vi "Save Copy of Cal Coefficients.vi"() -> ()   [LabVIEW 2016]
uses:
  Miscellaneous/Globals.vi
panel:
  out "Spreadsheet":string[][](array[string])
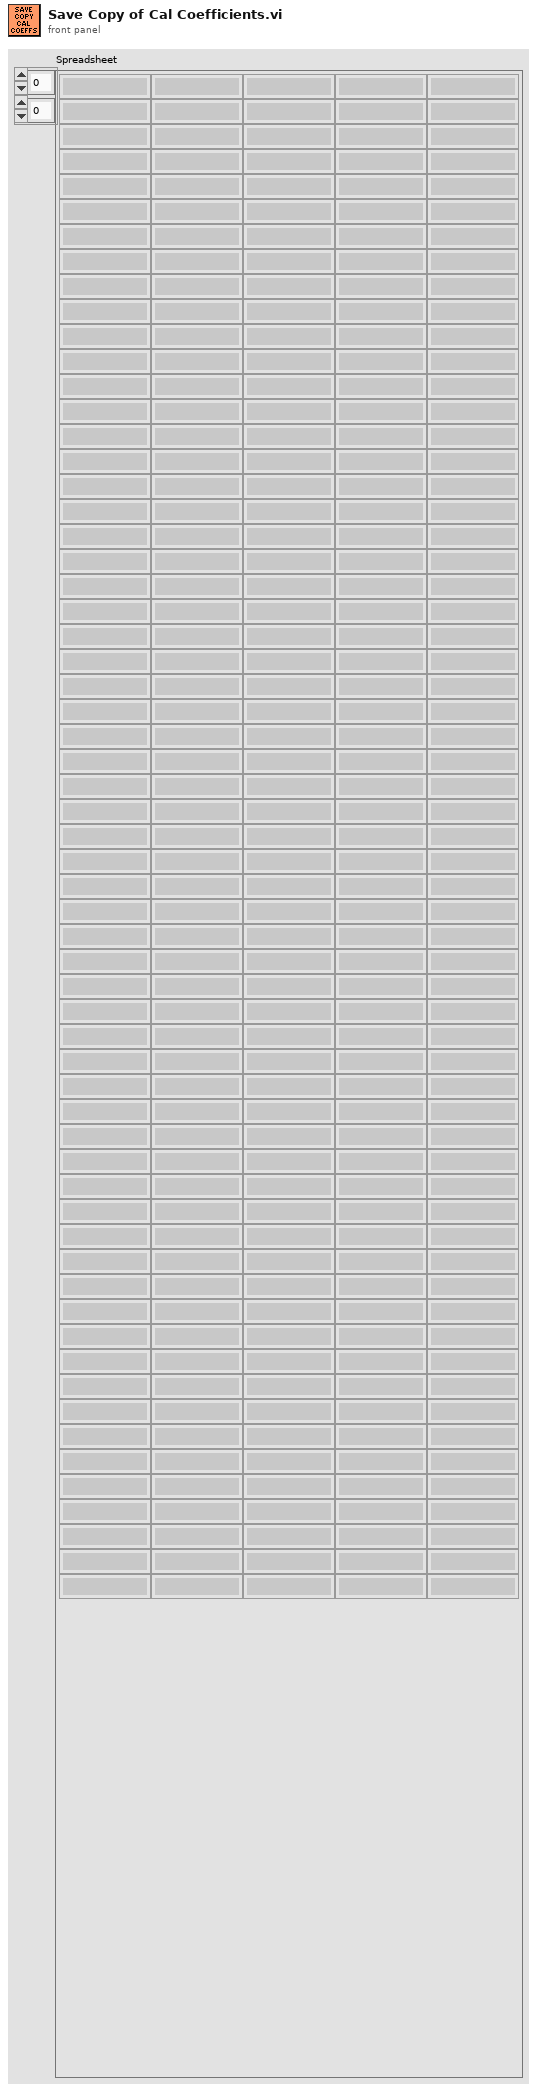
[diagram p1: front panel]
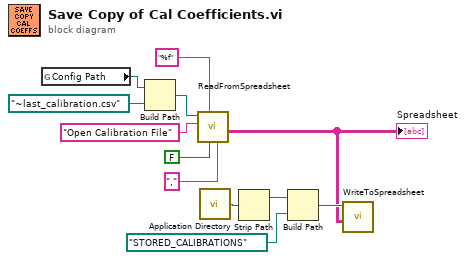
[diagram p0: block diagram]
diagram:
  n1 = global read "Globals.vi" "Config Path"() -> (w4:path)
  n2 = Build Path(base path=w4, name or relative path=path "~last_calibration.csv" ("Calfile")) -> (appended path=w9:path)
  n3 = call "ReadFromSpreadsheet.vi"("delimiter (\\t)"="," ("delimiter (\\t)"), "transpose (no:F)"=FALSE, "format (%d)"="%f", "File Prompt"="Open Calibration File", "file path"=w9) -> ("text array"=w5:string[][])  [unwired: 2 in, 4 out]
  "Spreadsheet" <- w5
  n4 = call <vilib>:"Application Directory.vi"() -> ("Application Directory"=w2:path)
  n5 = Strip Path(path=w2) -> (stripped path=w1:path)  [unwired: 1 out]
  n6 = Build Path(base path=w1, name or relative path=path "STORED_CALIBRATIONS" ("Calfile")) -> (appended path=w6:path)
  n7 = call "WriteToSpreadsheet.vi"("Spreadsheet"=w5, "file (use dialog)"=w6) -> ()  [unwired: 9 in, 1 out]
